vi "inversione senso di rotazione(SubVI).vi"(6 "Boolean in 2":bool, 7 "VersoOrarioM1":bool, 9 "Boolean in 1":bool) -> (0 "Boolean out 2":bool, 3 "Boolean out 1":bool)   [LabVIEW 2017]
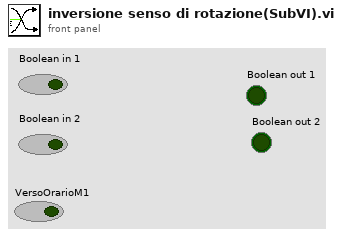
[diagram p1: front panel]
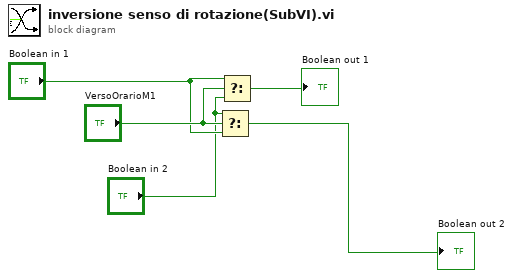
[diagram p0: block diagram]
diagram:
  n1 = Select(t="Boolean in 2", s="VersoOrarioM1", f="Boolean in 1") -> (s? t:f=→"Boolean out 2":bool)
  n2 = Select(t="Boolean in 1", s="VersoOrarioM1", f="Boolean in 2") -> (s? t:f=→"Boolean out 1":bool)
